vi "Set Server Key File.vi"(10 "Server Key File (.key)":path, 11 "OOP Server in":refnum<class "HVC8.lvclass">) -> (3 "OOP Server out":refnum<class "HVC8.lvclass">)   [LabVIEW 2019, in "HVC8.lvlib" / "HVC8.lvclass"]
uses:
  HVC8.lvclass
  HVC8.lvclass/HVC8.ctl
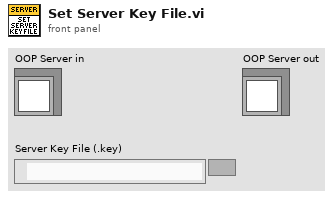
[diagram p1: front panel]
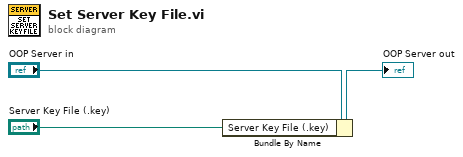
[diagram p0: block diagram]
diagram:
  n1 = Bundle By Name(cluster="OOP Server in", "Server Key File (.key)"="Server Key File (.key)") -> (→"OOP Server out":refnum<class "HVC8.lvclass">)
